vi "Init.vi"(8 "error in":errorcluster, 10 "Value":string, 11 "Value in":refnum<class "Value.lvclass">) -> (0 "error out":errorcluster, 3 "Value out":refnum<class "Value.lvclass">)   [LabVIEW 2019, in "Electronic Datasheet.lvlib" / "Value.lvclass"]
uses:
  Value.lvclass
  Value.lvclass/Value.ctl
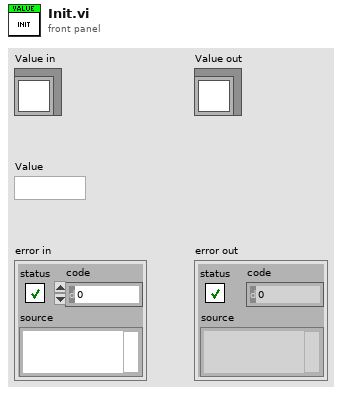
[diagram p1: front panel]
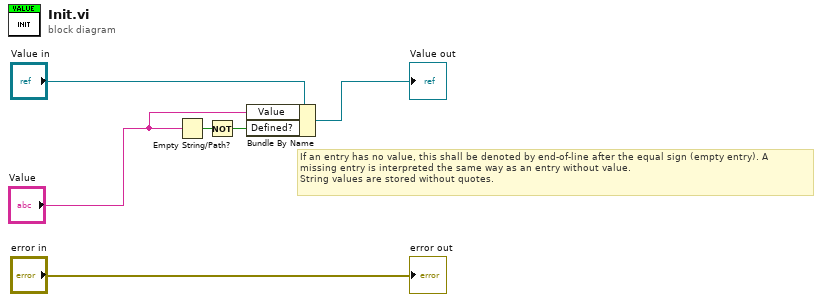
[diagram p0: block diagram]
diagram:
  # "If an entry has no value, this shall be denoted by end-of-line after the equal sign (empty entry). A \nmissing entry is interpreted the same way as an entry without value. \nString values are stored without quotes."
  n1 = Empty String/Path?(string/path="Value") -> (empty?=w3:bool)
  n2 = Not(x=w3) -> (.not. x?=w1:bool)
  n3 = Bundle By Name(cluster="Value in", "Value"="Value", "Defined?"=w1) -> (→"Value out":refnum<class "Value.lvclass">)
  "error out" <- "error in"
